vi "coordinate_errors.vi"(1 "reset":bool, 4 "error aux in (no error)":errorcluster, 5 "error in (no error)":errorcluster) -> (15 "status":bool, 19 "error":errorcluster)   [LabVIEW 2016]
doc: "For coordinating error conditions across parallel loops.\n\nProduced By:\n\n<B>Kod Integrations, LLC</B>\n4835 Marianne Drive\nMount Airy, MD 21771\nhttp://www.kodintegrations.com\nemail: info@kodintegrations.com\nphone: (240) 687-1288"
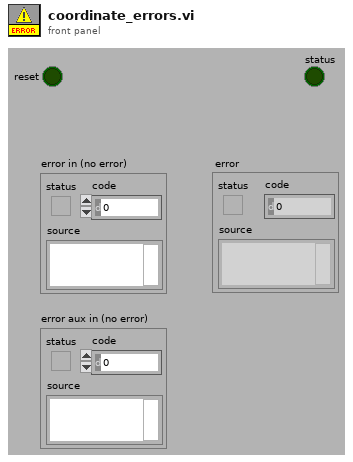
[diagram p1: front panel]
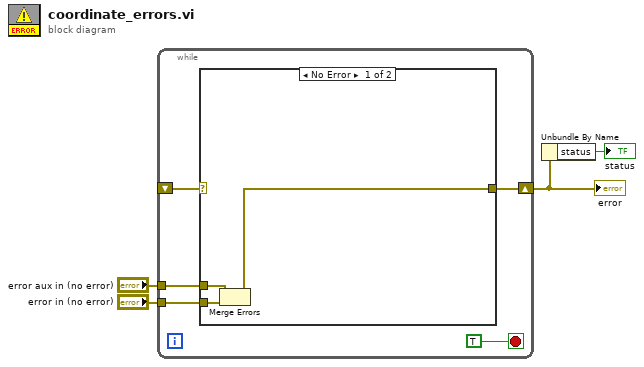
[diagram p0: block diagram]
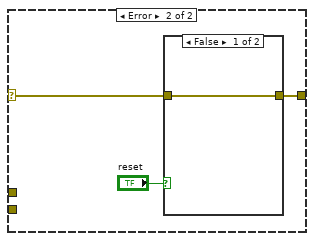
[diagram p2: hidden frame]
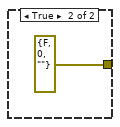
[diagram p3: hidden frame]
diagram:
  n1 = while {
    tunnel: "error in (no error)" -> [w7]
    shift-left: _ -> [w9]
    shift-right: [w8] -> w3
    tunnel: "error aux in (no error)" -> [w5]
    stop <- TRUE stop-if-true
    n2 = case shown="No Error" w9 {
      selector: w9 -> [_ w14]
      tunnel: [w10 w13] -> w8
      tunnel: w7 -> [w11 _]
      tunnel: w5 -> [w12 _]
      frame No Error {
        n3 = Merge Errors(w12, w11) -> (w10:errorcluster)
      }
      frame Error {
        n4 = case shown="False" "reset" {
          tunnel: w14 -> [w16 _]
          tunnel: [w16 errorcluster {"status"=FALSE, "code"=0, "source"=""} ("error IO")] -> w13
          frame False {
          }
          frame True {
          }
        }
      }
    }
  }
  "error" <- w3
  n5 = Unbundle By Name(w3) -> ("status"=→"status":bool)
